vi "Request Multiple Frames.vi"(8 "error in (no error)":errorcluster, 10 "Requests":T1[](array[typedef]), 11 "connection info":T2) -> (0 "error out":errorcluster, 2 "Response Frames":T4[](array[typedef]) {"payload" format="%x"; "timestamp" format="%<%.7X\n%x>T"; "type" items=["CAN Data"=0, "CAN Remote"=1, "CAN Bus Error"=2, "CAN 2.0 Data"=8, "CAN FD Data"=16, "CAN FD+BRS Data"=24, "J1939 Data"=192, "Delay"=224, "Log Trigger"=225, "Start Trigger"=226]; "identifier" format="%x"}, 3 "connection info":T2)   [LabVIEW 2015, in "J1939 Addon Shared.lvlib"]
uses:
  J1939 Addon Shared.lvlib
  <vilib>/xnet/xnet.llb/XNET Frame CAN.ctl
  <vilib>/xnet/xnet.llb/XNET Frame Type CAN.ctl
  <vilib>/NI/STM/TCP/TCP Connection Info.ctl
  <vilib>/NI/STM/SubVIs/MetaDataElement.ctl
  Types/Request Message.ctl
  <vilib>/NI/VeriStand Addon Network Comm/Shared/NI VeriStand Addon Network Comm Shared.lvlib
  <vilib>/NI/STM/NI STM.lvlib
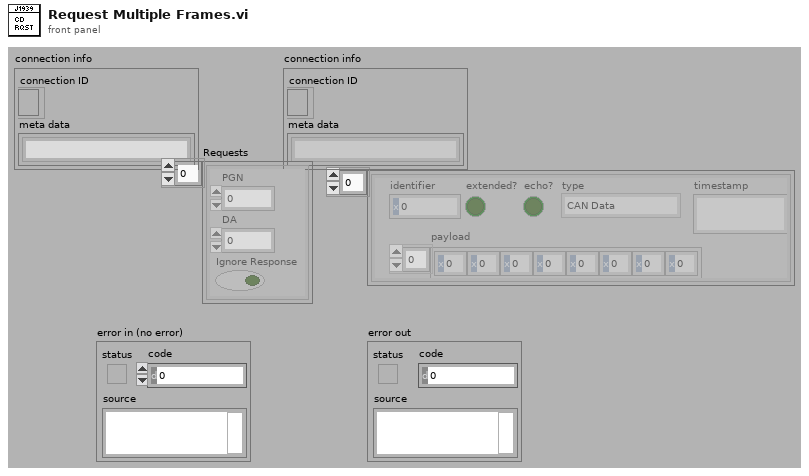
[diagram p1: front panel]
types:
  T1 = typedef "J1939 Addon Shared.lvlib/Request Message.ctl" = cluster{"PGN":u32, "DA":u8, "Ignore Response":bool}
  T2 = typedef "NI STM.lvlib/TCP Connection Info.ctl" = cluster{"connection ID":refnum<k5>, "meta data":T3[]}
  T3 = typedef "NI STM.lvlib/MetaDataElement.ctl" = string
  T4 = typedef "XNET Frame CAN.ctl" = cluster{"timestamp":timestamp, "payload":u8[], "identifier":u32, "type":T5, "extended?":bool, "echo?":bool}
  T5 = typedef "XNET Frame Type CAN.ctl" = u8
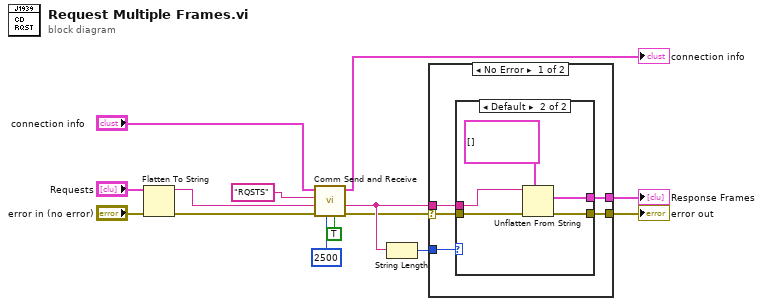
[diagram p0: block diagram]
diagram:
  n1 = Flatten To String(anything="Requests", error in (no error)="error in (no error)") -> (data string=w2:string, error out=w14:errorcluster)  [unwired: 2 in, 1 out]
  n2 = call <vilib>:"Comm Send and Receive.vi"("Resp Required?"=TRUE, "Timeout (ms)"=u32 2500 ("Timeout ms (5000)"), "error in (no error)"=w14, "Data"=w2, "Name"="RQSTS" ("Command"), "connection info"="connection info") -> ("error out"=w9:errorcluster, "Data"=w10:string, "connection info"=→"connection info":T2)  [unwired: 2 in, 1 out]
  n3 = String Length(string=w10) -> (length=w11:i32)
  n4 = case shown="No Error" w9 {
    selector: w9 -> [w16 w26]
    tunnel: [w19 w26] -> w5
    tunnel: w11 -> [w18 _]
    tunnel: w10 -> [w17 _]
    tunnel: [w15 _] -> w8
    frame No Error {
      n5 = case shown="Default" w18 {
        tunnel: w16 -> [w20 w25]
        tunnel: w17 -> [_ w21]
        tunnel: [w20 w24] -> w19
        tunnel: [_ w23] -> w15
        frame 0 {
        }
        frame Default {
          n6 = Unflatten From String(type=T4[] [], binary string=w21, error in (no error)=w25) -> (value=w23:T4[], error out=w24:errorcluster)  [unwired: 2 in, 1 out]
        }
      }
    }
    frame Error {
    }
  }
  "Response Frames" <- w8
  "error out" <- w5
